vi "Format_Exponent.vi"(0 "Numeric":dbl format="%#_6e", 1 "Total Width":i32=18, 2 "Precision":i32=10, 3 "Exponent Width":i32=2, 4 "Use System Decimal Point":bool=TRUE) -> (5 "String":string="  0.0000000000E+00", 6 "Returned String Length":i32)   [LabVIEW 2021]
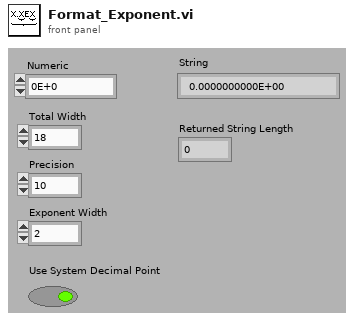
[diagram p1: front panel]
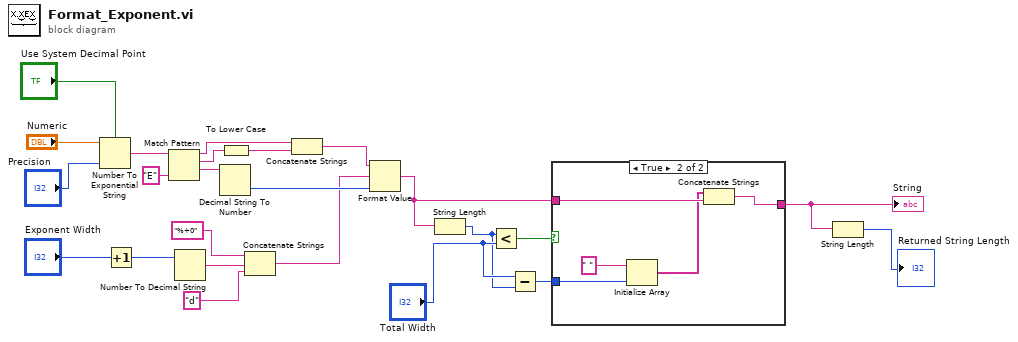
[diagram p0: block diagram]
diagram:
  n1 = Number To Exponential String(number="Numeric", precision (6)="Precision", 1:"Use System Decimal Point") -> (E-format string=w23:string)  [unwired: 1 in]
  n2 = Increment(x="Exponent Width") -> (x+1=w15:i32)
  n3 = Match Pattern(string=w23, regular expression="E") -> (before substring=w21:string, match substring=w2:string, after substring=w20:string)  [unwired: 1 in, 1 out]
  n4 = Number To Decimal String(number=w15) -> (decimal integer string=w13:string)  [unwired: 1 in]
  n5 = Decimal String To Number(string=w20) -> (number=w18:i32)  [unwired: 2 in, 1 out]
  n6 = To Lower Case(string=w2) -> (all lower case string=w1:string)
  n7 = Concatenate Strings("%+0", w13, "d") -> (w11:string)
  n8 = Concatenate Strings(w21, w1) -> (w19:string)
  n9 = Format Value(string ("")=w19, format string=w11, value (0)=w18) -> (output string=w6:string)
  n10 = String Length(string=w6) -> (length=w8:i32)
  n11 = Less?(x=w8, y="Total Width") -> (x < y?=w10:bool)
  n12 = Subtract(x="Total Width", y=w8) -> (x-y=w7:i32)
  n13 = case shown="True" w10 {
    tunnel: w7 -> [_ w29]
    tunnel: [w25 w28] -> w4
    tunnel: w6 -> [w25 w27]
    frame False {
    }
    frame True {
      n14 = Initialize Array(" ", w29) -> (w26:string[])
      n15 = Concatenate Strings(w26, w27) -> (w28:string)
    }
  }
  "String" <- w4
  n16 = String Length(string=w4) -> (length=→"Returned String Length":i32)
